vi "QSHelper(Unsigned Byte).vi"(8 "Indices In":i32[](array[numeric]), 9 "hi":i32, 10 "lo":i32, 11 "Array In":u8[](array[numeric])) -> (0 "Indices Out":i32[](array[numeric]), 3 "Array Out":u8[](array[numeric]))   [LabVIEW 2013, in "Sorting.lvlib"]
uses:
  Sorting.lvlib
  Partition Instances/Partition(Unsigned Byte).vi
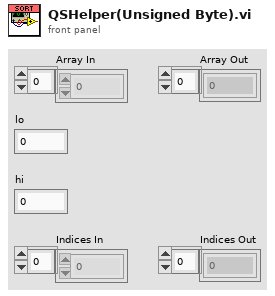
[diagram p1: front panel]
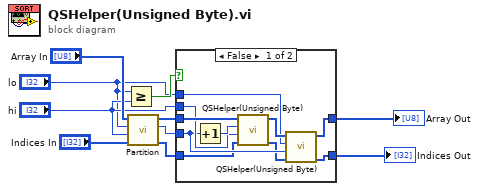
[diagram p0: block diagram]
diagram:
  n1 = Greater Or Equal?(x="lo", y="hi") -> (x >= y?=w9:bool)
  n2 = call-poly "Partition.vi"("Indices In"="Indices In", "hi"="hi", "lo"="lo", "Array In"="Array In") -> ("Indices Out"=w2:i32[], "pivot"=w6:i32, "Array Out"=w7:u8[])  [unwired: 5 in]
  n3 = case shown="False" w9 {
    tunnel: [w14 w22] -> w8
    tunnel: w7 -> [w20 w22]
    tunnel: w6 -> [w15 _]
    tunnel: "hi" -> [w18 _]
    tunnel: "lo" -> [w16 _]
    tunnel: w2 -> [w13 w21]
    tunnel: [w11 w21] -> w1
    frame False {
      n4 = Increment(x=w15) -> (x+1=w19:i32)
      n5 = call "QSHelper(Unsigned Byte).vi"("Indices In"=w13, "hi"=w18, "lo"=w19, "Array In"=w20) -> ("Indices Out"=w12:i32[], "Array Out"=w17:u8[])  [unwired: 6 in]
      n6 = call "QSHelper(Unsigned Byte).vi"("Indices In"=w12, "hi"=w15, "lo"=w16, "Array In"=w17) -> ("Indices Out"=w11:i32[], "Array Out"=w14:u8[])  [unwired: 6 in]
    }
    frame True {
    }
  }
  "Array Out" <- w8
  "Indices Out" <- w1
